vi "DualDigitalOscilloscopeTEST.vi"() -> ()   [LabVIEW 2014]
doc: "This digital oscilloscope requires a DAQ device\n\nSignal input to the ai0 port will produce a representation of the signal on the front panel. Triggering can be achieved by connecting the function generator's syn/ttl/trig out to the PFI 0 port on the DAQ device\n\nBryan Ghahremani -SID: 1135515\nKenneth Heide -SID: 1269429"
panel:
  out "error out":errorcluster
  in  "Digitizing Parameters":T1
  out "Waveform Graph":dynamicdata(graph)
  in  "stop":bool
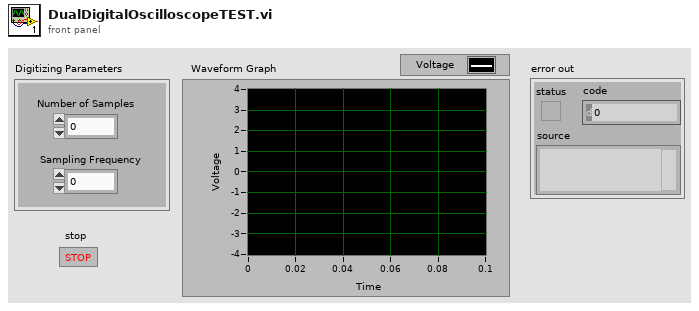
[diagram p1: front panel]
types:
  T1 = cluster{"Number of Samples":dbl, "Sampling Frequency":dbl}
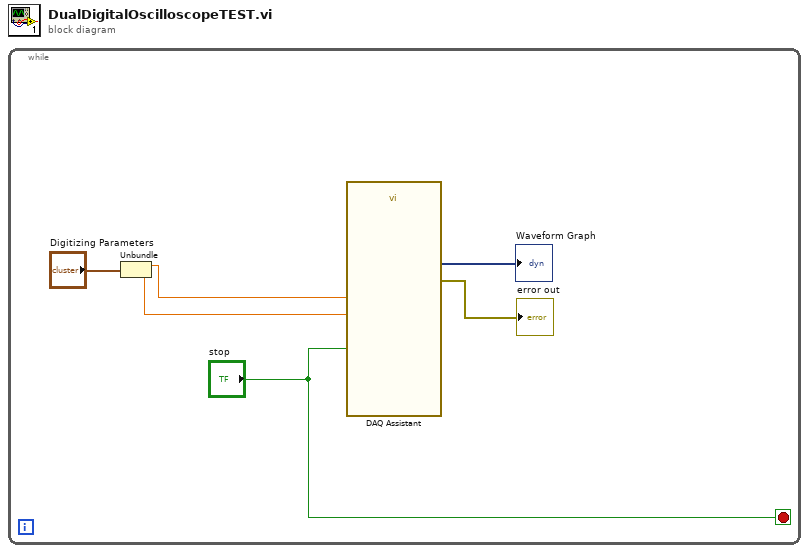
[diagram p0: block diagram]
diagram:
  n1 = while {
    stop <- "stop" stop-if-true
    n2 = Unbundle("Digitizing Parameters") -> ("Number of Samples"=w5:dbl, "Sampling Frequency"=w4:dbl)
    n3 = call "DAQ Assistant"("rate"=w4, "number of samples"=w5, "stop (T)"="stop") -> ("data"=→"Waveform Graph":dynamicdata, "error out"=→"error out":errorcluster)  [unwired: 14 in, 1 out]
  }
